vi "getDataFromJsonJobList.vi"(8 "errorIn":errorcluster, 10 "jobFileName":string, 11 "jobFilesFolderPath":path) -> (0 "errorOut":errorcluster, 3 "data":T1(array[cluster]))   [LabVIEW 2025]
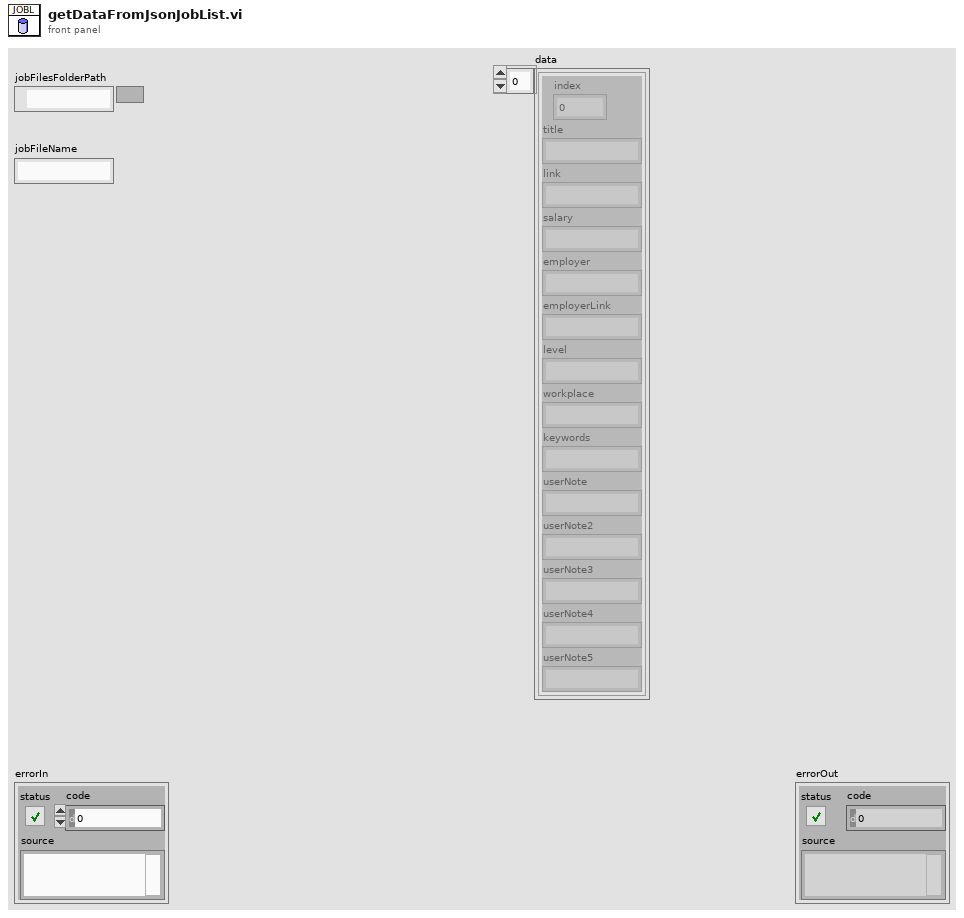
[diagram p1: front panel]
types:
  T1 = cluster{"index":i32, "title":string, "link":string, "salary":string, "employer":string, "employerLink":string, "level":string, "workplace":string, "keywords":string, "userNote":string, "userNote2":string, "userNote3":string, "userNote4":string, "userNote5":string}[]
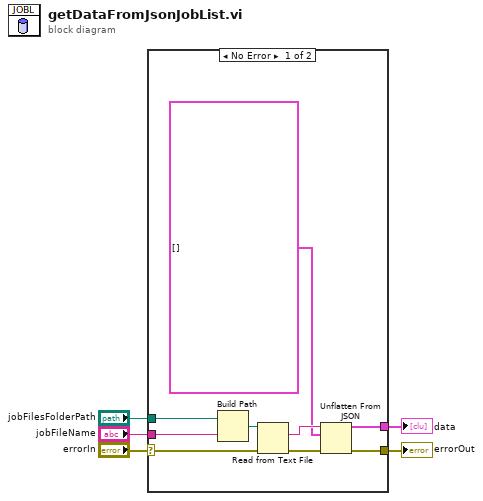
[diagram p0: block diagram]
diagram:
  n1 = case shown="No Error" "errorIn" {
    selector: "errorIn" -> [w7 w15]
    tunnel: "jobFileName" -> [w14 _]
    tunnel: [w13 w15] -> w4
    tunnel: "jobFilesFolderPath" -> [w12 _]
    tunnel: [w11 _] -> w1
    frame No Error {
      n2 = Build Path(base path=w12, name or relative path=w14) -> (appended path=w10:path)
      n3 = Read from Text File(file (use dialog)=w10, error in=w7) -> (text=w9:string, error out=w8:errorcluster)  [unwired: 2 in, 2 out]
      n4 = Unflatten From JSON(JSON string=w9, type and defaults=T1 [] ("template"), error in (no error)=w8) -> (value=w11:T1, error out=w13:errorcluster)  [unwired: 4 in]
    }
    frame Error {
    }
  }
  "errorOut" <- w4
  "data" <- w1
